vi "VisionSetGameStart.vi"(8 "Game Start":bool) -> ()   [LabVIEW 2020]
uses:
  VisionGlobal.vi
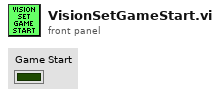
[diagram p1: front panel]
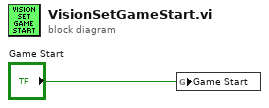
[diagram p0: block diagram]
diagram:
  n1 = global write "VisionGlobal.vi" "Game Start"("Game Start") -> ()
